vi "JTAG Test Setup.vi"(8 "error in (no error)":errorcluster, 9 "SET Value":u8, 10 "BIT Value":bool, 11 "Test Function":T1(ring)) -> (0 "error out":errorcluster)   [LabVIEW 2010]
panel:
  in  "Rev3+ Pluto?":bool=TRUE
  # "H"
  # "L"
  # "NOTE:  Offset shifting done automatically for SET values"
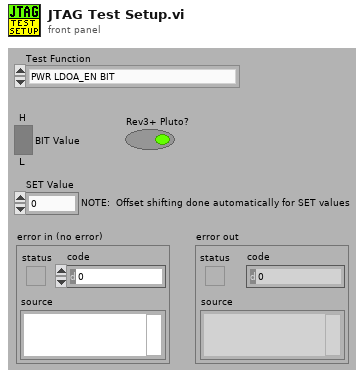
[diagram p1: front panel]
types:
  T1 = enum16{"PWR LDOA_EN BIT", "PWR VD1_EN BIT", "PWR VD2_EN BIT", "PWR VD3_EN BIT", "PWR VD4_EN BIT", "PWR BFG_EN BIT", "PWR TEMP_EN BIT", "PWR THERM_EN BIT", "PWR CHARGE_EN BIT", "PWR COMP_OV BIT", "PWR MSPBUF < MSPBUF_IN", "PWR MSPBUF < Fuel Gauge", "PWR MSPBUF < Recharge PM", "PWR MSPBUF < Temp_Out", "PWR MSPBUF < Therm_Bias", "PWR MSPBUF < Therm_Input", "PWR MSPBUF < Therm_Offset", "PWR MSPBUF OFF", "PWR ASK_POL BIT", "PWR MAGSW_DISABLE BIT", "PWR MAGTIME_SEL 00 (OFF)", "PWR MAGTIME_SEL 01 (5S)", "PWR MAGTIME_SEL 10 (2S)", "PWR MAGTIME_SEL 11 (TEST)", "PWR STROBE_INT_EN BIT", "PWR STROBE_PW SET", "PWR STROBE_FREQ SET", "PWR HCM_PW SET", "PWR LCM_DC SET"}
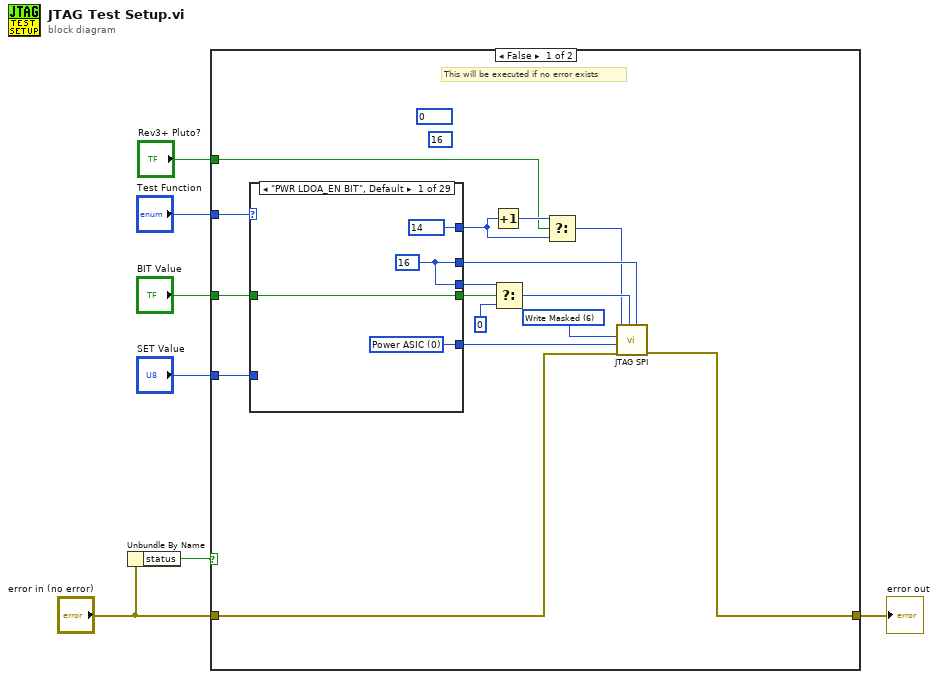
[diagram p0: block diagram]
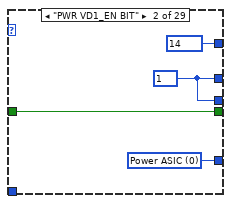
[diagram p2: hidden frame]
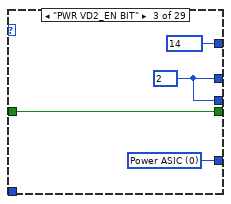
[diagram p3: hidden frame]
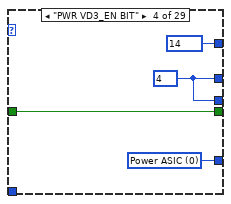
[diagram p4: hidden frame]
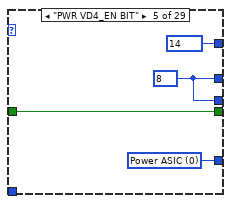
[diagram p5: hidden frame]
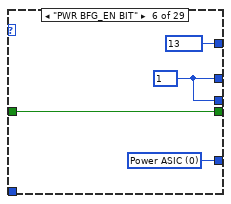
[diagram p6: hidden frame]
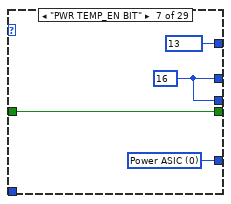
[diagram p7: hidden frame]
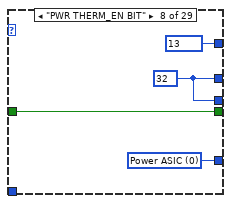
[diagram p8: hidden frame]
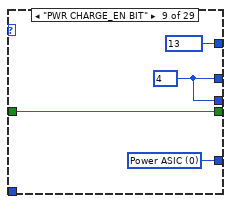
[diagram p9: hidden frame]
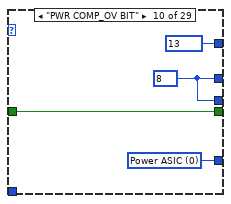
[diagram p10: hidden frame]
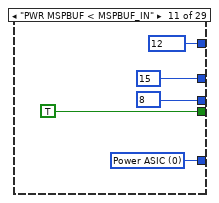
[diagram p11: hidden frame]
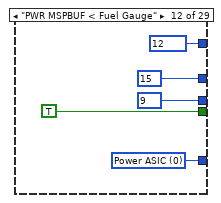
[diagram p12: hidden frame]
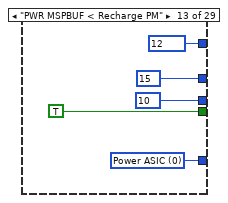
[diagram p13: hidden frame]
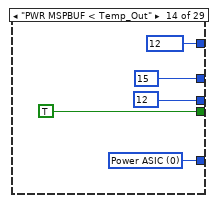
[diagram p14: hidden frame]
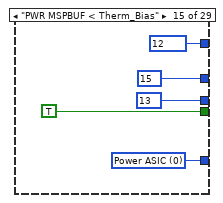
[diagram p15: hidden frame]
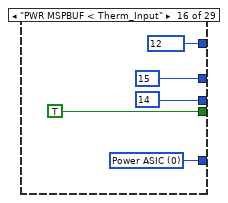
[diagram p16: hidden frame]
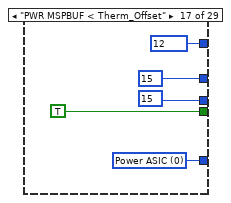
[diagram p17: hidden frame]
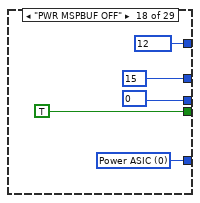
[diagram p18: hidden frame]
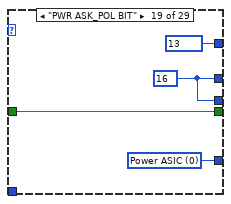
[diagram p19: hidden frame]
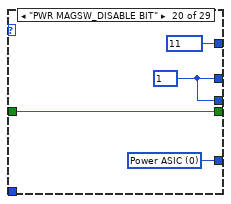
[diagram p20: hidden frame]
diagram:
  n1 = Unbundle By Name("error in (no error)") -> ("status"=w6:bool)
  n2 = case shown="False" w6 {
    tunnel: [w21 w160] -> w7
    tunnel: "error in (no error)" -> [w22 w160]
    tunnel: "Test Function" -> [w23 _]
    tunnel: "SET Value" -> [w15 _]
    tunnel: "BIT Value" -> [w13 _]
    tunnel: "Rev3+ Pluto?" -> [w8 _]
    frame False {
      (unwired) u8 16 ("Address")
      w18 = u16 6 items=["Power UP", "Power DN", "Write Single", "Read Single", "Write Block", "Read Block", "Write Masked", "Test Value"] ("Function")
      (unwired) u16 0 ("Address")
      # "This will be executed if no error exists"
      n3 = case shown="\"PWR LDOA_EN BIT\", Default" w23 {
        tunnel: [w25 w30 w35 w39 w43 w46 w49 w54 w57 w62 u8 15 ("Address") u8 15 ("Address") u8 15 ("Address") u8 15 ("Address") u8 15 ("Address") u8 15 ("Address") u8 15 ("Address") u8 15 ("Address") w105 w109 u8 6 ("Address") u8 6 ("Address") u8 6 ("Address") u8 6 ("Address") w134 u8 7 ("Address") u8 56 ("Address") u8 7 ("Address") u8 56 ("Address")] -> w20
        tunnel: [w27 w29 w33 w37 w41 w45 w50 w52 w56 w60 w65 w72 w77 w81 w86 w91 w95 w102 w107 w110 w116 w117 w122 w127 w133 w138 w144 w149 w154] -> w19
        tunnel: [w25 w30 w35 w39 w43 w46 w49 w54 w57 w62 u8 8 ("Address") u8 9 ("Address") u8 10 ("Address") u8 12 ("Address") u8 13 ("Address") u8 14 ("Address") u8 15 ("Address") u8 0 ("Address") w105 w109 u8 0 ("Address") u8 2 ("Address") u8 4 ("Address") u8 6 ("Address") w134 w136 w143 w148 w156] -> w17
        tunnel: [u16 14 ("Address") u16 14 ("Address") u16 14 ("Address") u16 14 ("Address") u16 14 ("Address") u16 13 ("Address") u16 13 ("Address") u16 13 ("Address") u16 13 ("Address") u16 13 ("Address") u16 12 ("Address") u16 12 ("Address") u16 12 ("Address") u16 12 ("Address") u16 12 ("Address") u16 12 ("Address") u16 12 ("Address") u16 12 ("Address") u16 13 ("Address") u16 11 ("Address") u16 11 ("Address") u16 11 ("Address") u16 11 ("Address") u16 11 ("Address") u16 14 ("Address") u16 15 ("Address") u16 15 ("Address") u16 16 ("Address") u16 15 ("Address")] -> w10
        tunnel: w15 -> [_ _ _ _ _ _ _ _ _ _ _ _ _ _ _ _ _ _ _ _ _ _ _ _ _ w136 w142 w148 w153]
        tunnel: [w24 w28 w32 w36 w40 w44 w51 w55 w59 w61 TRUE TRUE TRUE TRUE TRUE TRUE TRUE TRUE w104 w111 TRUE TRUE TRUE TRUE w132 TRUE TRUE TRUE TRUE] -> w14
        tunnel: w13 -> [w24 w28 w32 w36 w40 w44 w51 w55 w59 w61 _ _ _ _ _ _ _ _ w104 w111 _ _ _ _ w132 _ _ _ _]
        frame "PWR LDOA_EN BIT", Default {
          w27 = u16 0 items=["Power ASIC", "Stim ASIC", "MICS Radio", "FRAM"] ("Target")
          w25 = u8 16 ("Address")
        }
        frame "PWR VD1_EN BIT" {
          w29 = u16 0 items=["Power ASIC", "Stim ASIC", "MICS Radio", "FRAM"] ("Target")
          w30 = u8 1 ("Address")
        }
        frame "PWR VD2_EN BIT" {
          w33 = u16 0 items=["Power ASIC", "Stim ASIC", "MICS Radio", "FRAM"] ("Target")
          w35 = u8 2 ("Address")
        }
        frame "PWR VD3_EN BIT" {
          w37 = u16 0 items=["Power ASIC", "Stim ASIC", "MICS Radio", "FRAM"] ("Target")
          w39 = u8 4 ("Address")
        }
        frame "PWR VD4_EN BIT" {
          w41 = u16 0 items=["Power ASIC", "Stim ASIC", "MICS Radio", "FRAM"] ("Target")
          w43 = u8 8 ("Address")
        }
        frame "PWR BFG_EN BIT" {
          w45 = u16 0 items=["Power ASIC", "Stim ASIC", "MICS Radio", "FRAM"] ("Target")
          w46 = u8 1 ("Address")
        }
        frame "PWR TEMP_EN BIT" {
          w50 = u16 0 items=["Power ASIC", "Stim ASIC", "MICS Radio", "FRAM"] ("Target")
          w49 = u8 16 ("Address")
        }
        frame "PWR THERM_EN BIT" {
          w52 = u16 0 items=["Power ASIC", "Stim ASIC", "MICS Radio", "FRAM"] ("Target")
          w54 = u8 32 ("Address")
        }
        frame "PWR CHARGE_EN BIT" {
          w56 = u16 0 items=["Power ASIC", "Stim ASIC", "MICS Radio", "FRAM"] ("Target")
          w57 = u8 4 ("Address")
        }
        frame "PWR COMP_OV BIT" {
          w60 = u16 0 items=["Power ASIC", "Stim ASIC", "MICS Radio", "FRAM"] ("Target")
          w62 = u8 8 ("Address")
        }
        frame "PWR MSPBUF < MSPBUF_IN" {
          w65 = u16 0 items=["Power ASIC", "Stim ASIC", "MICS Radio", "FRAM"] ("Target")
        }
        frame "PWR MSPBUF < Fuel Gauge" {
          w72 = u16 0 items=["Power ASIC", "Stim ASIC", "MICS Radio", "FRAM"] ("Target")
        }
        frame "PWR MSPBUF < Recharge PM" {
          w77 = u16 0 items=["Power ASIC", "Stim ASIC", "MICS Radio", "FRAM"] ("Target")
        }
        frame "PWR MSPBUF < Temp_Out" {
          w81 = u16 0 items=["Power ASIC", "Stim ASIC", "MICS Radio", "FRAM"] ("Target")
        }
        frame "PWR MSPBUF < Therm_Bias" {
          w86 = u16 0 items=["Power ASIC", "Stim ASIC", "MICS Radio", "FRAM"] ("Target")
        }
        frame "PWR MSPBUF < Therm_Input" {
          w91 = u16 0 items=["Power ASIC", "Stim ASIC", "MICS Radio", "FRAM"] ("Target")
        }
        frame "PWR MSPBUF < Therm_Offset" {
          w95 = u16 0 items=["Power ASIC", "Stim ASIC", "MICS Radio", "FRAM"] ("Target")
        }
        frame "PWR MSPBUF OFF" {
          w102 = u16 0 items=["Power ASIC", "Stim ASIC", "MICS Radio", "FRAM"] ("Target")
        }
        frame "PWR ASK_POL BIT" {
          w107 = u16 0 items=["Power ASIC", "Stim ASIC", "MICS Radio", "FRAM"] ("Target")
          w105 = u8 16 ("Address")
        }
        frame "PWR MAGSW_DISABLE BIT" {
          w110 = u16 0 items=["Power ASIC", "Stim ASIC", "MICS Radio", "FRAM"] ("Target")
          w109 = u8 1 ("Address")
        }
        frame "PWR MAGTIME_SEL 00 (OFF)" {
          w116 = u16 0 items=["Power ASIC", "Stim ASIC", "MICS Radio", "FRAM"] ("Target")
        }
        frame "PWR MAGTIME_SEL 01 (5S)" {
          w117 = u16 0 items=["Power ASIC", "Stim ASIC", "MICS Radio", "FRAM"] ("Target")
        }
        frame "PWR MAGTIME_SEL 10 (2S)" {
          w122 = u16 0 items=["Power ASIC", "Stim ASIC", "MICS Radio", "FRAM"] ("Target")
        }
        frame "PWR MAGTIME_SEL 11 (TEST)" {
          w127 = u16 0 items=["Power ASIC", "Stim ASIC", "MICS Radio", "FRAM"] ("Target")
        }
        frame "PWR STROBE_INT_EN BIT" {
          w133 = u16 0 items=["Power ASIC", "Stim ASIC", "MICS Radio", "FRAM"] ("Target")
          w134 = u8 32 ("Address")
        }
        frame "PWR STROBE_PW SET" {
          w138 = u16 0 items=["Power ASIC", "Stim ASIC", "MICS Radio", "FRAM"] ("Target")
        }
        frame "PWR STROBE_FREQ SET" {
          w144 = u16 0 items=["Power ASIC", "Stim ASIC", "MICS Radio", "FRAM"] ("Target")
          n4 = Logical Shift(y=i8 3, x=w142) -> (x << y=w143:u8)
        }
        frame "PWR HCM_PW SET" {
          w149 = u16 0 items=["Power ASIC", "Stim ASIC", "MICS Radio", "FRAM"] ("Target")
        }
        frame "PWR LCM_DC SET" {
          w154 = u16 0 items=["Power ASIC", "Stim ASIC", "MICS Radio", "FRAM"] ("Target")
          n5 = Logical Shift(y=i8 3, x=w153) -> (x << y=w156:u8)
        }
      }
      n6 = Increment(x=w10) -> (x+1=w9:u16)
      n7 = Select(t=w17, s=w14, f=u8 0) -> (s? t:f=w16:u8)
      n8 = Select(t=w9, s=w8, f=w10) -> (s? t:f=w11:u16)
      n9 = call "JTAG SPI.vi"("Mask"=w20, "Value"=w16, "error in (no error)"=w22, "Target"=w19, "Function"=w18, "Address"=w11) -> ("error out"=w21:errorcluster)  [unwired: 2 in, 3 out]
    }
    frame True {
      # "Error exists, skip all functions"
    }
  }
  "error out" <- w7
